vi "Validate Variable Header.vi"(8 "error in (no error)":errorcluster, 11 "CONNACK in":refnum<class "CONNACK.lvclass">) -> (0 "error out":errorcluster, 1 "valid?":bool, 3 "CONNACK out":refnum<class "CONNACK.lvclass">)   [LabVIEW 2013, in "CONNACK.lvclass"]
uses:
  CONNACK.lvclass
  ControlPacket/ControlPacket.lvclass/ControlPacket.ctl
  ControlPacket/ControlPacket.lvclass
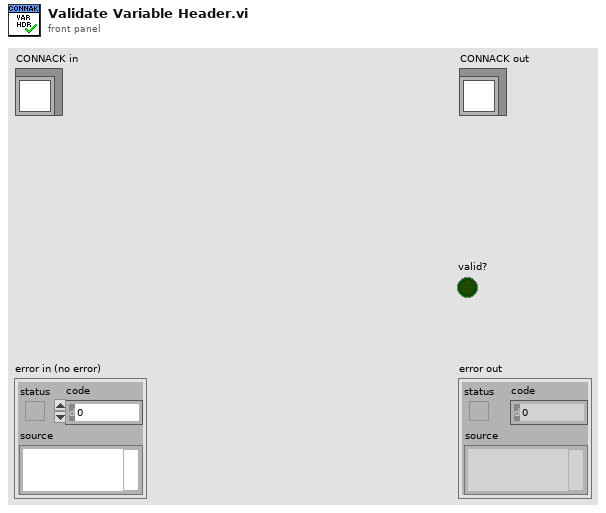
[diagram p1: front panel]
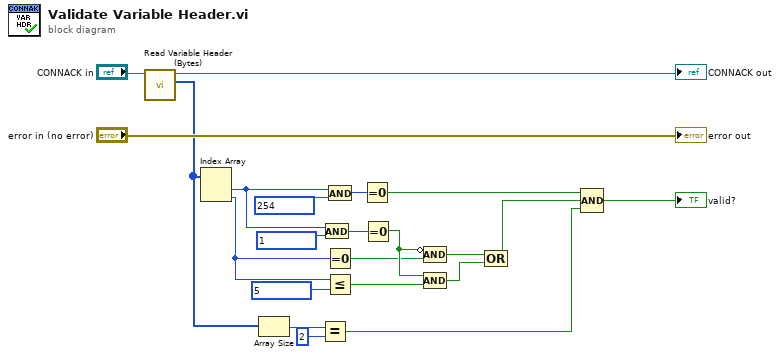
[diagram p0: block diagram]
diagram:
  n1 = call "Read Variable Header (Bytes).vi"("ControlPacket in"="CONNACK in") -> ("Variable Header (Bytes)"=w1:u8[], "ControlPacket out"=→"CONNACK out":refnum<class "CONNACK.lvclass">)  [unwired: 9 in]
  n2 = Index Array(array=w1) -> (element #1=w12:u8, element #2=w6:u8)  [unwired: 2 in]
  n3 = Array Size(array=w1) -> (size(s)=w20:i32)
  n4 = Equal?(x=w20, y=2) -> (x = y?=w18:bool)
  n5 = And(x=w12, y=u8 1) -> (x .and. y?=w7:u8)
  n6 = And(x=w12, y=u8 254) -> (x .and. y?=w21:u8)
  n7 = Equal To 0?(x=w6) -> (x = 0?=w5:bool)
  n8 = Less Or Equal?(x=w6, y=u8 5) -> (x <= y?=w4:bool)
  n9 = Equal To 0?(x=w21) -> (x = 0?=w11:bool)
  n10 = Equal To 0?(x=w7) -> (x = 0?=w8:bool)
  n11 = Compound Arithmetic op=AND(invert w8, w5) -> (w9:bool)
  n12 = Compound Arithmetic op=AND(w8, w4) -> (w3:bool)
  n13 = Compound Arithmetic op=OR(w9, w3) -> (w2:bool)
  n14 = Compound Arithmetic op=AND(w11, w2, w18) -> (→"valid?":bool)
  "error out" <- "error in (no error)"
